vi "BRig_RT_panel_ExpStruct_v1,18.vi"(7 "input_setValues":bool, 11 "input_dataExp":u16[](array[numeric])) -> (3 "output_dataExp":u16[](array[numeric]))   [LabVIEW 2014]
panel:
  in  "DAB_flipLR_nTrial_opt":bool caption="Rewards\n\nTrials"
  in  "DAB_flipLR_nTrial":u16=100 caption="Flip Directionality\nAfter X trials" max=1000 step=1
  in  "I_L_nTrig_PerState":bool
  in  "I_Cue2":bool caption="Enable Cue2?\n\n\nENL2\n\nCue2 Audio\nCue2 LED"
  in  "T_Cue2_LED_max":u16=1000 caption="Max" min=5 max=5000 step=5
  in  "T_Cue2_LED_min":u16=1000 caption="Min" min=5 max=5000 step=5
  in  "T_Cue2_LED_step":u16=1000 caption="Penalty" min=1 max=10000 step=1
  in  "T_Cue2_Audio_max":u16=1000 caption="Max" min=5 max=5000 step=5
  in  "T_Cue2_Audio_min":u16=1000 caption="Min" min=5 max=5000 step=5
  in  "T_Cue2_Audio_step":u16=1000 caption="Penalty" min=1 max=10000 step=1
  in  "T_ENL2_step":u16=100 caption="Penalty" min=10 max=10000 step=10
  in  "T_ENL2_max":u16=1000 caption="Max" min=250 max=10000 step=250
  in  "T_ENL2_min":u16=1000 caption="Min" min=250 max=10000 step=250
  in  "ClosedLoop_LaserHold_l2":bool
  in  "ClosedLoop_LaserHold_l1":bool
  in  "FreeReward_Count2":u16 caption="# consecutive NonForcedError trials"
  in  "FreeReward_Count1":u16 caption="# consecutive ReBiasing trials"
  in  "FreeReward_Switch":bool caption="Give Reward If\nToo Many Errors"
  in  "T_CuePenalty":u16=1000 caption="Penalty" min=1 max=10000 step=1
  in  "T_ENLPenalty":u16=100 caption="Penalty" min=10 max=10000 step=10
  in  "LaserSwitch_Probability_L1":u16
  in  "LaserSwitch":u16(slide) max=3 step=1 scale=0.0..3.0
  in  "I_DAB":bool caption="NonSpecific\nLick Direction"
  in  "Tcycle_Reward_max_R":u16=1000 caption="Max" min=5 max=5000 step=5
  in  "Tcycle_Reward_min_R":u16=1000 caption="Min" min=5 max=5000 step=5
  in  "Tcycle_Reward_step_R":u16=1000 caption="Penalty" min=1 max=10000 step=1
  in  "Tcycle_Reward_max_L":u16=1000 caption="Max" min=5 max=5000 step=5
  in  "Tcycle_Reward_min_L":u16=1000 caption="Min" min=5 max=5000 step=5
  in  "Tcycle_Reward_step_L":u16=1000 caption="Penalty" min=1 max=10000 step=1
  in  "T_Cue_LED_max":u16=1000 caption="Max" min=5 max=5000 step=5
  in  "T_Cue_LED_min":u16=1000 caption="Min" min=5 max=5000 step=5
  in  "T_Cue_LED_step":u16=1000 caption="Penalty" min=1 max=10000 step=1
  in  "SolenoidProbability_L":u16=100 caption="Reward Time [ms]" min=1 max=1000 step=1
  in  "SolenoidProbability_R":u16=100 caption="Reward Time [ms]" min=1 max=1000 step=1
  in  "T_Cue_Audio_max":u16=1000 caption="Max" min=5 max=5000 step=5
  in  "T_Cue_Audio_min":u16=1000 caption="Min" min=5 max=5000 step=5
  in  "BUR_max":u16 caption="Max"
  in  "Tcycle_Timeout":u16=1000 caption="Timeout Time [ms]" min=10 max=10000 step=1
  in  "Tcycle_Wrong":u16=1000 caption="Penalty - Wrong Choice" min=10 max=10000 step=1
  in  "Tcycle_Selection":u16=1000 caption="Answer Time [ms]" min=1 max=10000 step=1
  in  "Tcycle_RewardPost":u16=1000 caption="Consumption Time [ms]" min=250 max=10000 step=250
  in  "TpB_Max_R":u16=4 caption="Max R" min=1 max=12 step=1
  in  "TpB_Min_R":u16=4 caption="Min R" min=1 max=12 step=1
  in  "TpB_Max_L":u16=4 caption="Max L" min=1 max=12 step=1
  in  "TpB_Min_L":u16=4 caption="Min L" min=1 max=12 step=1
  in  "BUR_min":u16 caption="Min"
  in  "TrialUntilReward":bool caption="Ignore Wrong\nSelections?"
  in  "T_Cue_Audio_step":u16=1000 caption="Penalty" min=1 max=10000 step=1
  in  "T_ENL_step":u16=100 caption="Penalty" min=10 max=10000 step=10
  in  "T_ENL_max":u16=1000 caption="Max" min=250 max=10000 step=250
  in  "T_ENL_min":u16=1000 caption="Min" min=250 max=10000 step=250
  # "Experiment Task Structure"
  # "Min            Max               Step        Penalty"
  # "(Laser1 or Laser2)\nLaser1 probability"
  # "Enforced\nNonLick"
  # "Cue Audio"
  # "(ClosedLoop Structure)"
  # "Hold Laser1"
  # "Hold Laser2"
  # "Cue LED"
  # "Allow Multiple Laser\nTriggers During\nENL and Cue?"
  # "Dual Armed Bandit"
  # "Selection"
  # "Reward - Dispense Water"
  # "Min            Max            StepSize"
  # "Left"
  # "Right"
  # "Count Reward Structure\n(0 = off)"
  # "Dispense Water Probability"
  # "%"
  # "Left"
  # "Right"
  # "%"
  # "Trial Per Block Structure \n               Left                        Right"
  # "Reward - Consumption"
  # "Penalty - Choice Timeout"
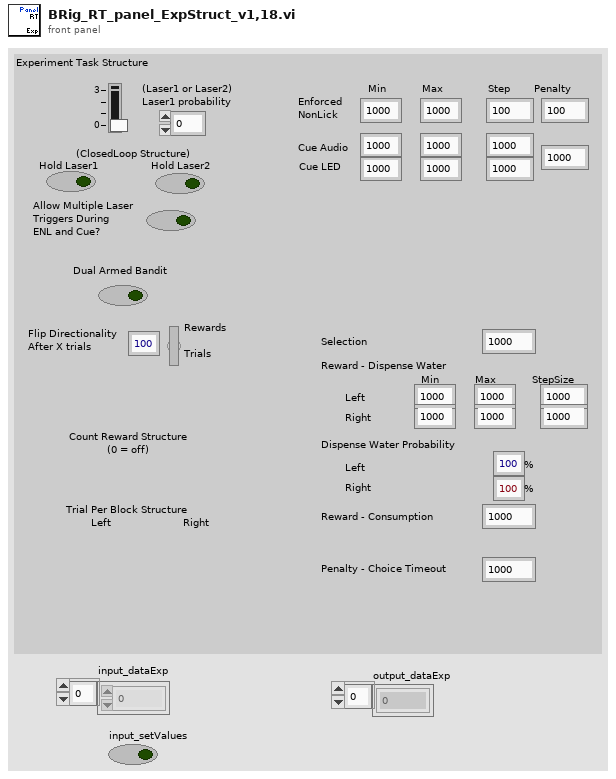
[diagram p1: front panel]
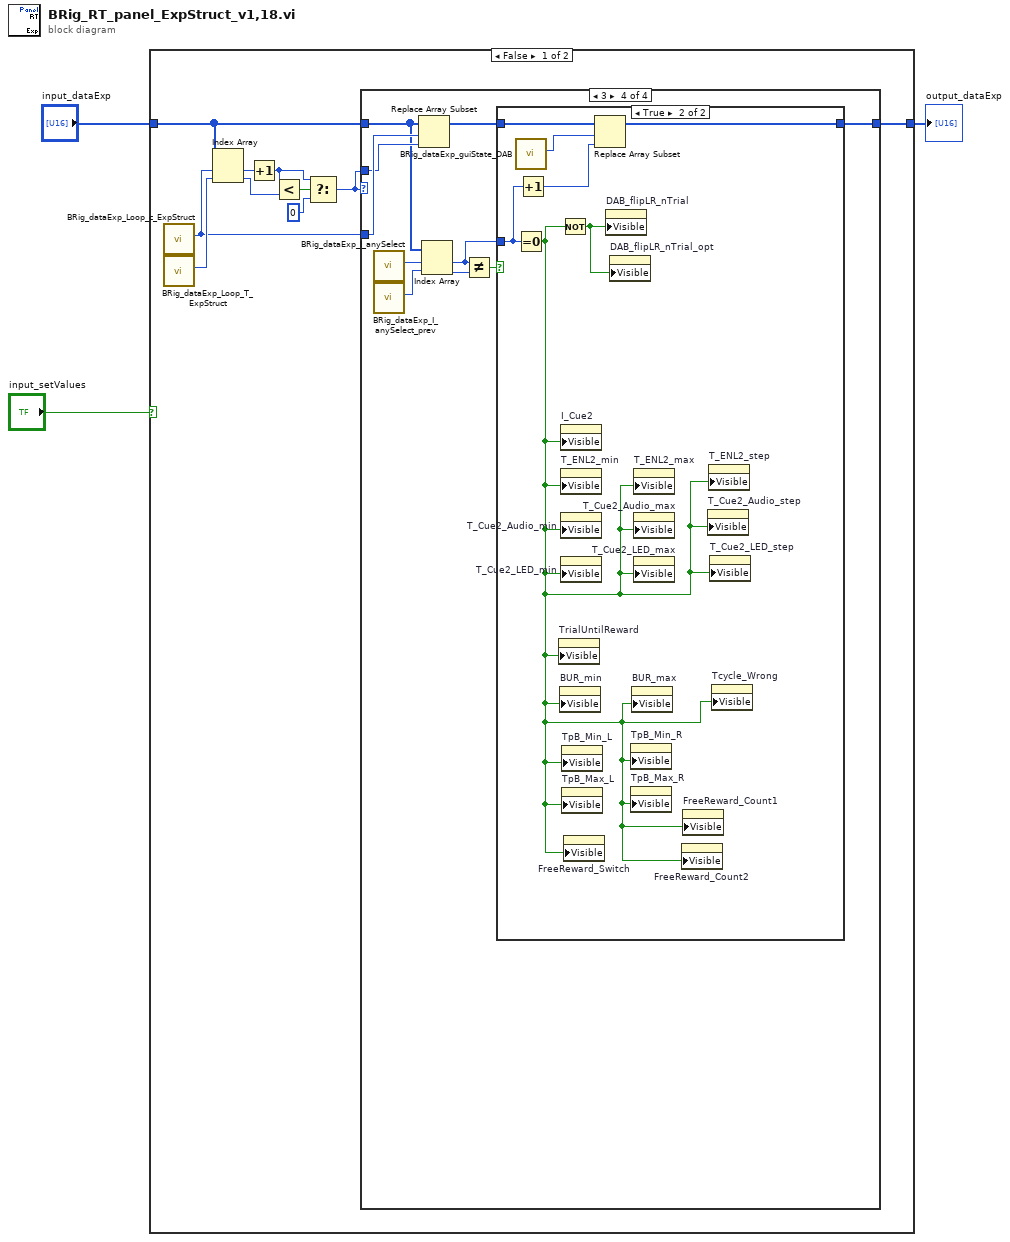
[diagram p0: block diagram]
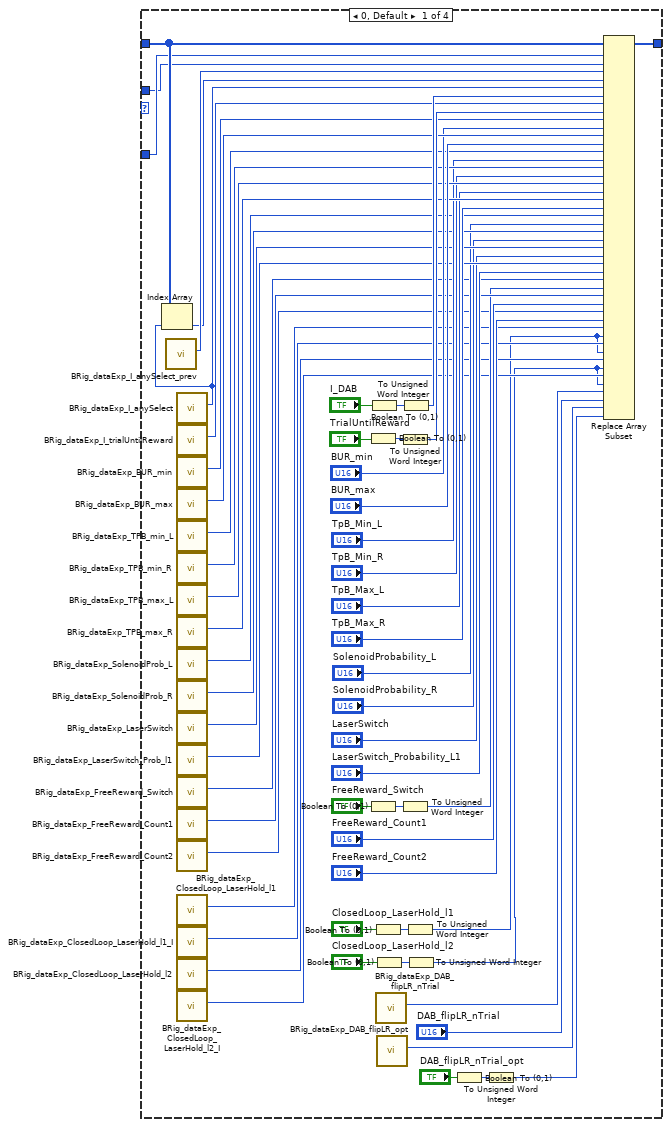
[diagram p2: hidden frame]
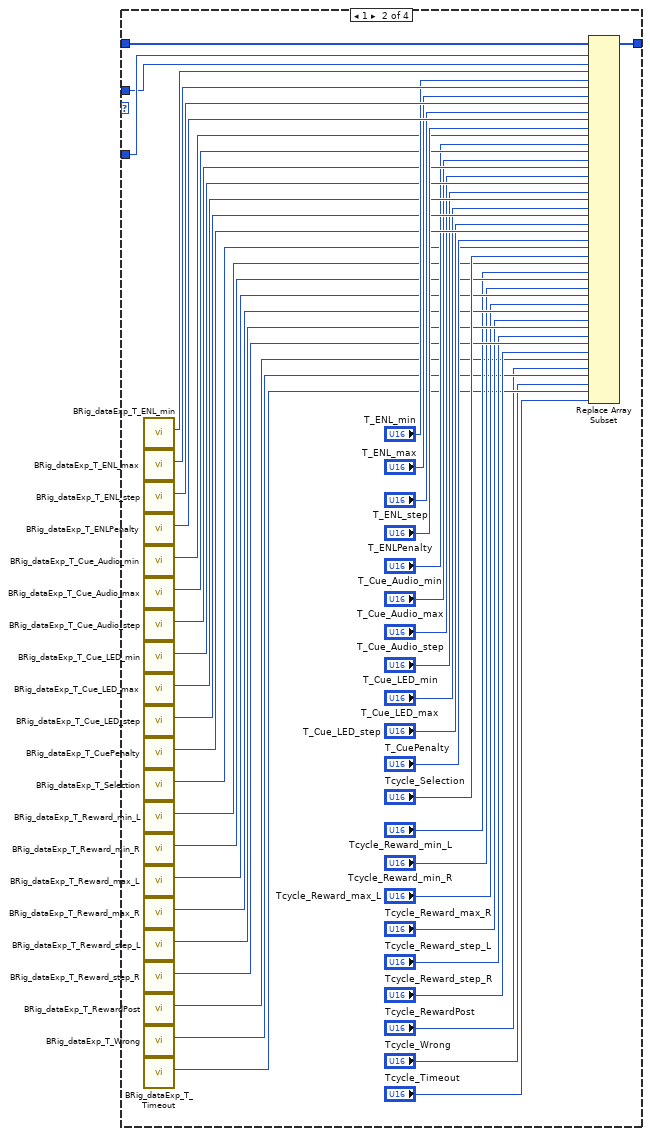
[diagram p3: hidden frame]
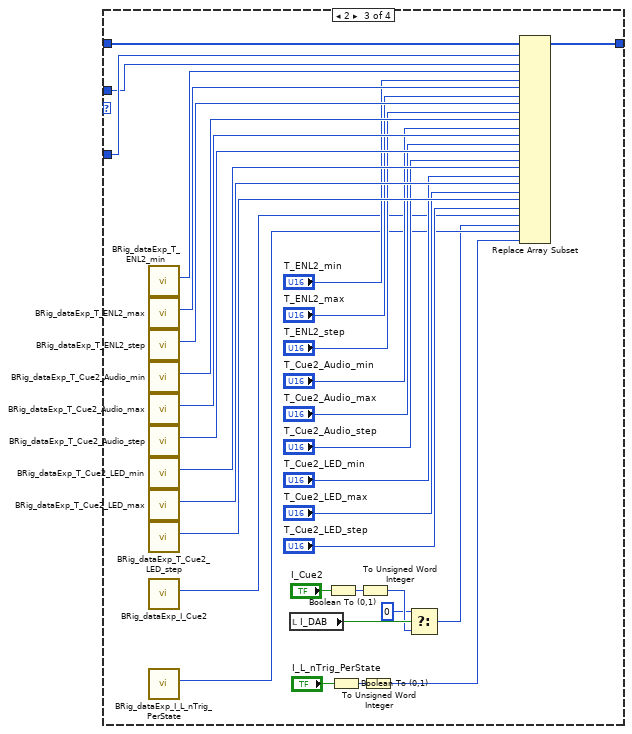
[diagram p4: hidden frame]
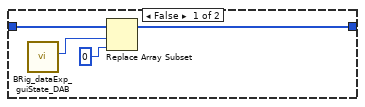
[diagram p5: hidden frame]
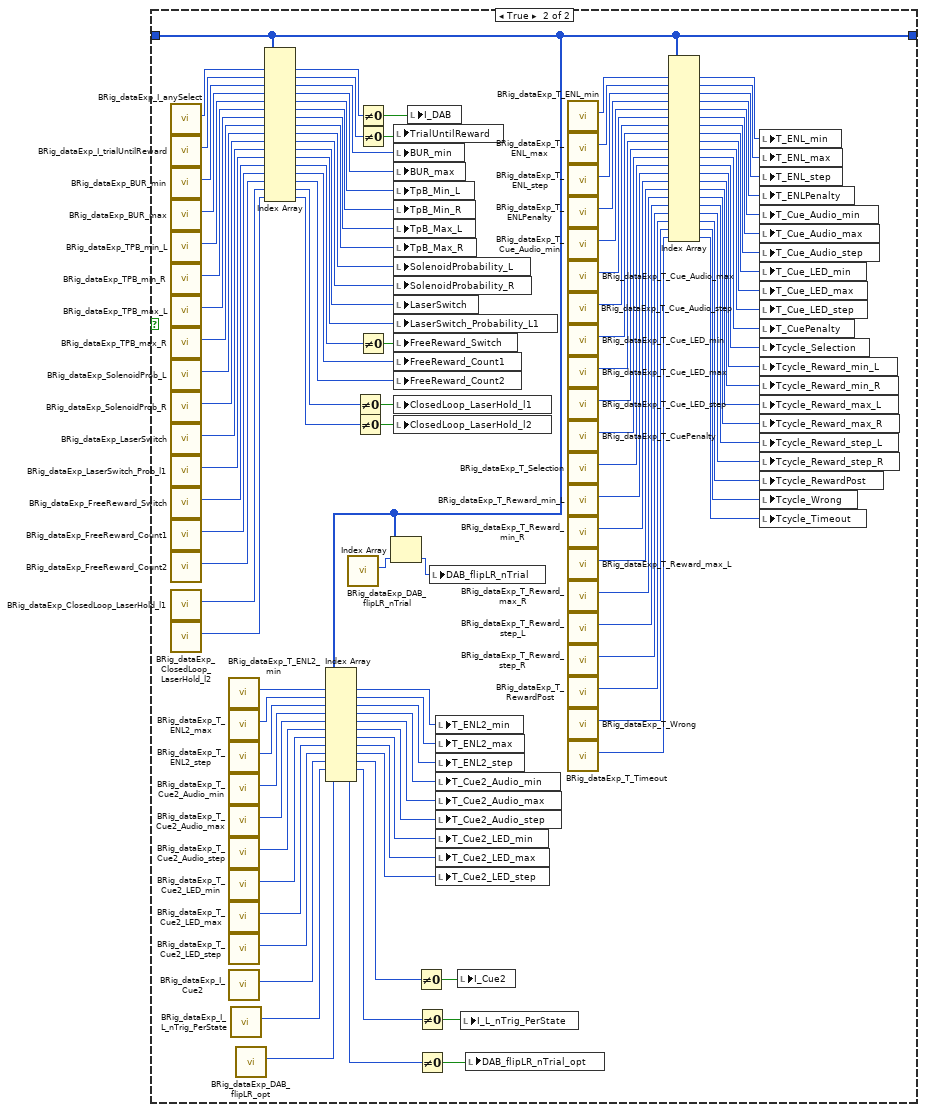
[diagram p6: hidden frame]
diagram:
  n1 = case shown="False" "input_setValues" {
    tunnel: [w13 w177] -> w3
    tunnel: "input_dataExp" -> [w12 w177]
    frame False {
      n2 = call "BRig_dataExp_Loop_c_ExpStruct.vi"() -> ("output_Loop_c_ExpStruct"=w6:i32)  [unwired: 11 in]
      n3 = call "BRig_dataExp_Loop_T_ExpStruct.vi"() -> ("output_Loop_T_ExpStruct"=w11:i32)  [unwired: 11 in]
      n4 = Index Array(array=w12, index #1=w6, index #2=w11) -> (element #1=w10:u16, element #2=w9:u16)
      n5 = Increment(x=w10) -> (x+1=w5:u16)
      n6 = Less?(x=w5, y=w9) -> (x < y?=w8:bool)
      n7 = Select(t=w5, s=w8, f=u16 0) -> (s? t:f=w4:u16)
      n8 = case shown="3" w4 {
        tunnel: w12 -> [w23 w117 w150 w157]
        tunnel: [w71 w116 w149 w152] -> w13
        tunnel: w6 -> [w21 w115 w148 w160]
        tunnel: w4 -> [w20 w114 w147 w159]
        frame 0, Default {
          n9 = call "BRig_dataExp_I_anySelect_prev.vi"() -> ("output_I_anySelect_prev"=w19:i32)  [unwired: 11 in]
          n10 = call "BRig_dataExp_I_anySelect.vi"() -> ("output_I_anySelect"=w22:i32)  [unwired: 11 in]
          n11 = Index Array(array=w23, index=w22) -> (element=w18:u16)
          n12 = call "BRig_dataExp_I_trialUntilReward.vi"() -> ("output_I_trialUntilReward"=w67:i32)  [unwired: 11 in]
          n13 = call "BRig_dataExp_BUR_min.vi"() -> ("output_BUR_min"=w63:i32)  [unwired: 11 in]
          n14 = call "BRig_dataExp_BUR_max.vi"() -> ("output_BUR_max"=w62:i32)  [unwired: 11 in]
          n15 = call "BRig_dataExp_TPB_min_L.vi"() -> ("output_TPB_min_L"=w59:i32)  [unwired: 11 in]
          n16 = call "BRig_dataExp_TPB_min_R.vi"() -> ("output_TPB_min_R"=w58:i32)  [unwired: 11 in]
          n17 = call "BRig_dataExp_TPB_max_L.vi"() -> ("output_TPB_max_L"=w57:i32)  [unwired: 11 in]
          n18 = call "BRig_dataExp_TPB_max_R.vi"() -> ("output_TPB_max_R"=w56:i32)  [unwired: 11 in]
          n19 = call "BRig_dataExp_SolenoidProb_L.vi"() -> ("output_SolenoidProbability_L"=w51:i32)  [unwired: 11 in]
          n20 = call "BRig_dataExp_SolenoidProb_R.vi"() -> ("output_SolenoidProbability_R"=w50:i32)  [unwired: 11 in]
          n21 = call "BRig_dataExp_LaserSwitch.vi"() -> ("output_LaserSwitch"=w49:i32)  [unwired: 11 in]
          n22 = call "BRig_dataExp_LaserSwitch_Prob_l1.vi"() -> ("output_LaserSwitch_Probability_L1"=w48:i32)  [unwired: 11 in]
          n23 = call "BRig_dataExp_FreeReward_Switch.vi"() -> ("output_FreeReward_Switch"=w41:i32)  [unwired: 11 in]
          n24 = call "BRig_dataExp_FreeReward_Count1.vi"() -> ("output_FreeReward_Count"=w40:i32)  [unwired: 11 in]
          n25 = call "BRig_dataExp_FreeReward_Count2.vi"() -> ("output_FreeReward_Count"=w37:i32)  [unwired: 11 in]
          n26 = call "BRig_dataExp_ClosedLoop_LaserHold_l1.vi"() -> ("output_CloseLoop_LaserHold_l1"=w35:i32)  [unwired: 11 in]
          n27 = call "BRig_dataExp_ClosedLoop_LaserHold_l1_I.vi"() -> ("output_CloseLoop_LaserHold_l1_I"=w34:i32)  [unwired: 11 in]
          n28 = call "BRig_dataExp_ClosedLoop_LaserHold_l2.vi"() -> ("output_CloseLoop_LaserHold_l2"=w33:i32)  [unwired: 11 in]
          n29 = call "BRig_dataExp_ClosedLoop_LaserHold_l2_I.vi"() -> ("output_CloseLoop_LaserHold_l2_I"=w32:i32)  [unwired: 11 in]
          n30 = Boolean To (0,1)(Boolean="TrialUntilReward") -> (0, 1=w66:i16)
          n31 = Boolean To (0,1)(Boolean="FreeReward_Switch") -> (0, 1=w43:i16)
          n32 = Boolean To (0,1)(Boolean="I_DAB") -> (0, 1=w69:i16)
          n33 = Boolean To (0,1)(Boolean="ClosedLoop_LaserHold_l1") -> (0, 1=w31:i16)
          n34 = Boolean To (0,1)(Boolean="ClosedLoop_LaserHold_l2") -> (0, 1=w29:i16)
          n35 = call "BRig_dataExp_DAB_flipLR_nTrial.vi"() -> ("output_DAB_flipLR_nTrial"=w25:i32)  [unwired: 11 in]
          n36 = call "BRig_dataExp_DAB_flipLR_opt.vi"() -> ("output_DAB_flipLR_opt"=w17:i32)  [unwired: 11 in]
          n37 = To Unsigned Word Integer(number=w66) -> (unsigned 16bit integer=w64:u16)
          n38 = To Unsigned Word Integer(number=w43) -> (unsigned 16bit integer=w39:u16)
          n39 = To Unsigned Word Integer(number=w69) -> (unsigned 16bit integer=w68:u16)
          n40 = To Unsigned Word Integer(number=w31) -> (unsigned 16bit integer=w27:u16)
          n41 = To Unsigned Word Integer(number=w29) -> (unsigned 16bit integer=w26:u16)
          n42 = Boolean To (0,1)(Boolean="DAB_flipLR_nTrial_opt") -> (0, 1=w16:i16)
          n43 = To Unsigned Word Integer(number=w16) -> (unsigned 16bit integer=w14:u16)
          n44 = Replace Array Subset(array=w23, new element #1=w20, index #1=w21, new element #2=w18, index #2=w19, new element #3=w68, index #3=w22, new element #4=w64, index #4=w67, new element #5="BUR_min", index #5=w63, new element #6="BUR_max", index #6=w62, new element #7="TpB_Min_L", index #7=w59, new element #8="TpB_Min_R", index #8=w58, new element #9="TpB_Max_L", index #9=w57, new element #10="TpB_Max_R", index #10=w56, new element #11="SolenoidProbability_L", index #11=w51, new element #12="SolenoidProbability_R", index #12=w50, new element #13="LaserSwitch", index #13=w49, new element #14="LaserSwitch_Probability_L1", index #14=w48, new element #15=w39, index #15=w41, new element #16="FreeReward_Count1", index #16=w40, new element #17="FreeReward_Count2", index #17=w37, new element #18=w27, index #18=w35, new element #19=w27, index #19=w34, new element #20=w26, index #20=w33, new element #21=w26, index #21=w32, new element #22="DAB_flipLR_nTrial", index #22=w25, new element #23=w14, index #23=w17) -> (w71:u16[])
        }
        frame 1 {
          n45 = call "BRig_dataExp_T_ENL_min.vi"() -> ("output_T_ENL_min"=w113:i32)  [unwired: 11 in]
          n46 = call "BRig_dataExp_T_ENL_max.vi"() -> ("output_T_ENL_max"=w112:i32)  [unwired: 11 in]
          n47 = call "BRig_dataExp_T_ENL_step.vi"() -> ("output_T_ENL_step"=w111:i32)  [unwired: 11 in]
          n48 = call "BRig_dataExp_T_ENLPenalty.vi"() -> ("output_ENL_penalty"=w110:i32)  [unwired: 11 in]
          n49 = call "BRig_dataExp_T_Cue_Audio_min.vi"() -> ("output_T_Cue_Audio_min"=w105:i32)  [unwired: 11 in]
          n50 = call "BRig_dataExp_T_Cue_Audio_max.vi"() -> ("output_T_Cue_Audio_max"=w104:i32)  [unwired: 11 in]
          n51 = call "BRig_dataExp_T_Cue_Audio_step.vi"() -> ("output_T_Cue_Audio_step"=w103:i32)  [unwired: 11 in]
          n52 = call "BRig_dataExp_T_Cue_LED_min.vi"() -> ("output_T_Cue_LED_min"=w102:i32)  [unwired: 11 in]
          n53 = call "BRig_dataExp_T_Cue_LED_max.vi"() -> ("output_T_Cue_LED_max"=w101:i32)  [unwired: 11 in]
          n54 = call "BRig_dataExp_T_Cue_LED_step.vi"() -> ("output_T_Cue_LED_step"=w100:i32)  [unwired: 11 in]
          n55 = call "BRig_dataExp_T_CuePenalty.vi"() -> ("output_T_CuePenalty"=w99:i32)  [unwired: 11 in]
          n56 = call "BRig_dataExp_T_Selection.vi"() -> ("output_T_Selection"=w91:i32)  [unwired: 11 in]
          n57 = call "BRig_dataExp_T_Reward_min_L.vi"() -> ("output_Tcycle_Reward_min_L"=w89:i32)  [unwired: 11 in]
          n58 = call "BRig_dataExp_T_Reward_min_R.vi"() -> ("output_T_Reward_min_R"=w88:i32)  [unwired: 11 in]
          n59 = call "BRig_dataExp_T_Reward_max_L.vi"() -> ("output_T_Reward_max_L"=w87:i32)  [unwired: 11 in]
          n60 = call "BRig_dataExp_T_Reward_max_R.vi"() -> ("output_T_Reward_max_R"=w86:i32)  [unwired: 11 in]
          n61 = call "BRig_dataExp_T_Reward_step_L.vi"() -> ("output_T_Reward_step_L"=w85:i32)  [unwired: 11 in]
          n62 = call "BRig_dataExp_T_Reward_step_R.vi"() -> ("output_T_Reward_step_R"=w84:i32)  [unwired: 11 in]
          n63 = call "BRig_dataExp_T_RewardPost.vi"() -> ("output_T_RewardPost"=w77:i32)  [unwired: 11 in]
          n64 = call "BRig_dataExp_T_Wrong.vi"() -> ("output_T_Wrong"=w76:i32)  [unwired: 11 in]
          n65 = call "BRig_dataExp_T_Timeout.vi"() -> ("output_T_Timeout"=w75:i32)  [unwired: 11 in]
          n66 = Replace Array Subset(array=w117, new element #1=w114, index #1=w115, new element #2="T_ENL_min", index #2=w113, new element #3="T_ENL_max", index #3=w112, new element #4="T_ENL_step", index #4=w111, new element #5="T_ENLPenalty", index #5=w110, new element #6="T_Cue_Audio_min", index #6=w105, new element #7="T_Cue_Audio_max", index #7=w104, new element #8="T_Cue_Audio_step", index #8=w103, new element #9="T_Cue_LED_min", index #9=w102, new element #10="T_Cue_LED_max", index #10=w101, new element #11="T_Cue_LED_step", index #11=w100, new element #12="T_CuePenalty", index #12=w99, new element #13="Tcycle_Selection", index #13=w91, new element #14="Tcycle_Reward_min_L", index #14=w89, new element #15="Tcycle_Reward_min_R", index #15=w88, new element #16="Tcycle_Reward_max_L", index #16=w87, new element #17="Tcycle_Reward_max_R", index #17=w86, new element #18="Tcycle_Reward_step_L", index #18=w85, new element #19="Tcycle_Reward_step_R", index #19=w84, new element #20="Tcycle_RewardPost", index #20=w77, new element #21="Tcycle_Wrong", index #21=w76, new element #22="Tcycle_Timeout", index #22=w75) -> (w116:u16[])
        }
        frame 2 {
          n67 = call "BRig_dataExp_T_ENL2_min.vi"() -> ("output_T_ENL2_min"=w146:i32)  [unwired: 11 in]
          n68 = call "BRig_dataExp_T_ENL2_max.vi"() -> ("output_T_ENL2_max"=w145:i32)  [unwired: 11 in]
          n69 = call "BRig_dataExp_T_ENL2_step.vi"() -> ("output_T_ENL2_step"=w144:i32)  [unwired: 11 in]
          n70 = call "BRig_dataExp_T_Cue2_Audio_min.vi"() -> ("output_T_Cue2_Audio_min"=w143:i32)  [unwired: 11 in]
          n71 = call "BRig_dataExp_T_Cue2_Audio_max.vi"() -> ("output_T_Cue2_Audio_max"=w142:i32)  [unwired: 11 in]
          n72 = call "BRig_dataExp_T_Cue2_Audio_step.vi"() -> ("output_T_Cue2_Audio_step"=w141:i32)  [unwired: 11 in]
          n73 = call "BRig_dataExp_T_Cue2_LED_min.vi"() -> ("output_T_Cue2_LED_min"=w140:i32)  [unwired: 11 in]
          n74 = call "BRig_dataExp_T_Cue2_LED_max.vi"() -> ("output_T_Cue2_LED_max"=w139:i32)  [unwired: 11 in]
          n75 = call "BRig_dataExp_T_Cue2_LED_step.vi"() -> ("output_T_Cue2_LED_step"=w138:i32)  [unwired: 11 in]
          n76 = call "BRig_dataExp_I_Cue2.vi"() -> ("output_I_Cue2"=w128:i32)  [unwired: 11 in]
          n77 = call "BRig_dataExp_I_L_nTrig_PerState.vi"() -> ("output_I_L_nTrig_PerState"=w125:i32)  [unwired: 11 in]
          n78 = local read "I_DAB"() -> (w121:bool)
          n79 = Boolean To (0,1)(Boolean="I_Cue2") -> (0, 1=w126:i16)
          n80 = Boolean To (0,1)(Boolean="I_L_nTrig_PerState") -> (0, 1=w124:i16)
          n81 = To Unsigned Word Integer(number=w126) -> (unsigned 16bit integer=w119:u16)
          n82 = To Unsigned Word Integer(number=w124) -> (unsigned 16bit integer=w122:u16)
          n83 = Select(t=u16 0 ("f"), s=w121, f=w119) -> (s? t:f=w120:u16)
          n84 = Replace Array Subset(array=w150, new element #1=w147, index #1=w148, new element #2="T_ENL2_min", index #2=w146, new element #3="T_ENL2_max", index #3=w145, new element #4="T_ENL2_step", index #4=w144, new element #5="T_Cue2_Audio_min", index #5=w143, new element #6="T_Cue2_Audio_max", index #6=w142, new element #7="T_Cue2_Audio_step", index #7=w141, new element #8="T_Cue2_LED_min", index #8=w140, new element #9="T_Cue2_LED_max", index #9=w139, new element #10="T_Cue2_LED_step", index #10=w138, new element #11=w120, index #11=w128, new element #12=w122, index #12=w125) -> (w149:u16[])
        }
        frame 3 {
          n85 = call "BRig_dataExp_I_anySelect.vi"() -> ("output_I_anySelect"=w158:i32)  [unwired: 11 in]
          n86 = call "BRig_dataExp_I_anySelect_prev.vi"() -> ("output_I_anySelect_prev"=w156:i32)  [unwired: 11 in]
          n87 = Replace Array Subset(array=w157, new element=w159, index=w160) -> (w153:u16[])
          n88 = Index Array(array=w157, index #1=w158, index #2=w156) -> (element #1=w151:u16, element #2=w155:u16)
          n89 = Not Equal?(x=w151, y=w155) -> (x != y?=w154:bool)
          n90 = case shown="True" w154 {
            tunnel: w153 -> [w164 w171]
            tunnel: [w163 w170] -> w152
            tunnel: w151 -> [_ w167]
            frame False {
              n91 = call "BRig_dataExp_guiState_DAB.vi"() -> ("output_guiState_DAB"=w162:i32)  [unwired: 11 in]
              n92 = Replace Array Subset(array=w164, new element=u16 0 ("new element/subarray"), index=w162) -> (w163:u16[])
            }
            frame True {
              n93 = call "BRig_dataExp_guiState_DAB.vi"() -> ("output_guiState_DAB"=w169:i32)  [unwired: 11 in]
              n94 = Equal To 0?(x=w167) -> (x = 0?=w166:bool)
              n95 = Increment(x=w167) -> (x+1=w168:u16)
              n96 = property on="TrialUntilReward" class="Bool (strict)"("Visible"=w166) -> ()  [unwired: 2 in, 2 out]
              n97 = Not(x=w166) -> (.not. x?=w165:bool)
              n98 = property on="BUR_min" class="DigNum (strict)"("Visible"=w166) -> ()  [unwired: 2 in, 2 out]
              n99 = property on="I_Cue2" class="Bool (strict)"("Visible"=w166) -> ()  [unwired: 2 in, 2 out]
              n100 = property on="T_ENL2_min" class="DigNum (strict)"("Visible"=w166) -> ()  [unwired: 2 in, 2 out]
              n101 = property on="T_Cue2_Audio_min" class="DigNum (strict)"("Visible"=w166) -> ()  [unwired: 2 in, 2 out]
              n102 = property on="T_Cue2_LED_min" class="DigNum (strict)"("Visible"=w166) -> ()  [unwired: 2 in, 2 out]
              n103 = property on="TpB_Min_L" class="DigNum (strict)"("Visible"=w166) -> ()  [unwired: 2 in, 2 out]
              n104 = property on="TpB_Max_L" class="DigNum (strict)"("Visible"=w166) -> ()  [unwired: 2 in, 2 out]
              n105 = property on="FreeReward_Switch" class="Bool (strict)"("Visible"=w166) -> ()  [unwired: 2 in, 2 out]
              n106 = Replace Array Subset(array=w171, new element=w168, index=w169) -> (w170:u16[])
              n107 = property on="DAB_flipLR_nTrial" class="DigNum (strict)"("Visible"=w165) -> ()  [unwired: 2 in, 2 out]
              n108 = property on="DAB_flipLR_nTrial_opt" class="Bool (strict)"("Visible"=w165) -> ()  [unwired: 2 in, 2 out]
              n109 = property on="TpB_Min_R" class="DigNum (strict)"("Visible"=w166) -> ()  [unwired: 2 in, 2 out]
              n110 = property on="TpB_Max_R" class="DigNum (strict)"("Visible"=w166) -> ()  [unwired: 2 in, 2 out]
              n111 = property on="BUR_max" class="DigNum (strict)"("Visible"=w166) -> ()  [unwired: 2 in, 2 out]
              n112 = property on="T_ENL2_max" class="DigNum (strict)"("Visible"=w166) -> ()  [unwired: 2 in, 2 out]
              n113 = property on="T_Cue2_Audio_max" class="DigNum (strict)"("Visible"=w166) -> ()  [unwired: 2 in, 2 out]
              n114 = property on="T_Cue2_LED_max" class="DigNum (strict)"("Visible"=w166) -> ()  [unwired: 2 in, 2 out]
              n115 = property on="FreeReward_Count2" class="DigNum (strict)"("Visible"=w166) -> ()  [unwired: 2 in, 2 out]
              n116 = property on="FreeReward_Count1" class="DigNum (strict)"("Visible"=w166) -> ()  [unwired: 2 in, 2 out]
              n117 = property on="T_Cue2_Audio_step" class="DigNum (strict)"("Visible"=w166) -> ()  [unwired: 2 in, 2 out]
              n118 = property on="T_ENL2_step" class="DigNum (strict)"("Visible"=w166) -> ()  [unwired: 2 in, 2 out]
              n119 = property on="T_Cue2_LED_step" class="DigNum (strict)"("Visible"=w166) -> ()  [unwired: 2 in, 2 out]
              n120 = property on="Tcycle_Wrong" class="DigNum (strict)"("Visible"=w166) -> ()  [unwired: 2 in, 2 out]
            }
          }
        }
      }
    }
    frame True {
      n121 = call "BRig_dataExp_I_anySelect.vi"() -> ("output_I_anySelect"=w282:i32)  [unwired: 11 in]
      n122 = call "BRig_dataExp_I_trialUntilReward.vi"() -> ("output_I_trialUntilReward"=w281:i32)  [unwired: 11 in]
      n123 = call "BRig_dataExp_BUR_min.vi"() -> ("output_BUR_min"=w280:i32)  [unwired: 11 in]
      n124 = call "BRig_dataExp_BUR_max.vi"() -> ("output_BUR_max"=w279:i32)  [unwired: 11 in]
      n125 = call "BRig_dataExp_TPB_min_L.vi"() -> ("output_TPB_min_L"=w278:i32)  [unwired: 11 in]
      n126 = call "BRig_dataExp_TPB_min_R.vi"() -> ("output_TPB_min_R"=w277:i32)  [unwired: 11 in]
      n127 = call "BRig_dataExp_TPB_max_L.vi"() -> ("output_TPB_max_L"=w276:i32)  [unwired: 11 in]
      n128 = call "BRig_dataExp_TPB_max_R.vi"() -> ("output_TPB_max_R"=w275:i32)  [unwired: 11 in]
      n129 = call "BRig_dataExp_SolenoidProb_L.vi"() -> ("output_SolenoidProbability_L"=w274:i32)  [unwired: 11 in]
      n130 = call "BRig_dataExp_SolenoidProb_R.vi"() -> ("output_SolenoidProbability_R"=w273:i32)  [unwired: 11 in]
      n131 = call "BRig_dataExp_LaserSwitch.vi"() -> ("output_LaserSwitch"=w272:i32)  [unwired: 11 in]
      n132 = call "BRig_dataExp_LaserSwitch_Prob_l1.vi"() -> ("output_LaserSwitch_Probability_L1"=w271:i32)  [unwired: 11 in]
      n133 = call "BRig_dataExp_FreeReward_Switch.vi"() -> ("output_FreeReward_Switch"=w270:i32)  [unwired: 11 in]
      n134 = call "BRig_dataExp_FreeReward_Count1.vi"() -> ("output_FreeReward_Count"=w269:i32)  [unwired: 11 in]
      n135 = call "BRig_dataExp_FreeReward_Count2.vi"() -> ("output_FreeReward_Count"=w209:i32)  [unwired: 11 in]
      n136 = call "BRig_dataExp_ClosedLoop_LaserHold_l1.vi"() -> ("output_CloseLoop_LaserHold_l1"=w207:i32)  [unwired: 11 in]
      n137 = call "BRig_dataExp_ClosedLoop_LaserHold_l2.vi"() -> ("output_CloseLoop_LaserHold_l2"=w206:i32)  [unwired: 11 in]
      n138 = call "BRig_dataExp_T_ENL2_min.vi"() -> ("output_T_ENL2_min"=w201:i32)  [unwired: 11 in]
      n139 = call "BRig_dataExp_T_ENL2_max.vi"() -> ("output_T_ENL2_max"=w200:i32)  [unwired: 11 in]
      n140 = call "BRig_dataExp_T_ENL2_step.vi"() -> ("output_T_ENL2_step"=w199:i32)  [unwired: 11 in]
      n141 = call "BRig_dataExp_T_Cue2_Audio_min.vi"() -> ("output_T_Cue2_Audio_min"=w198:i32)  [unwired: 11 in]
      n142 = call "BRig_dataExp_T_Cue2_Audio_max.vi"() -> ("output_T_Cue2_Audio_max"=w197:i32)  [unwired: 11 in]
      n143 = call "BRig_dataExp_T_Cue2_Audio_step.vi"() -> ("output_T_Cue2_Audio_step"=w196:i32)  [unwired: 11 in]
      n144 = call "BRig_dataExp_T_Cue2_LED_min.vi"() -> ("output_T_Cue2_LED_min"=w195:i32)  [unwired: 11 in]
      n145 = call "BRig_dataExp_T_Cue2_LED_max.vi"() -> ("output_T_Cue2_LED_max"=w194:i32)  [unwired: 11 in]
      n146 = call "BRig_dataExp_T_Cue2_LED_step.vi"() -> ("output_T_Cue2_LED_step"=w193:i32)  [unwired: 11 in]
      n147 = call "BRig_dataExp_I_Cue2.vi"() -> ("output_I_Cue2"=w183:i32)  [unwired: 11 in]
      n148 = call "BRig_dataExp_I_L_nTrig_PerState.vi"() -> ("output_I_L_nTrig_PerState"=w180:i32)  [unwired: 11 in]
      n149 = call "BRig_dataExp_DAB_flipLR_opt.vi"() -> ("output_DAB_flipLR_opt"=w174:i32)  [unwired: 11 in]
      n150 = Index Array(array=w177, index #1=w282, index #2=w281, index #3=w280, index #4=w279, index #5=w278, index #6=w277, index #7=w276, index #8=w275, index #9=w274, index #10=w273, index #11=w272, index #12=w271, index #13=w270, index #14=w269, index #15=w209, index #16=w207, index #17=w206) -> (element #1=w265:u16, element #2=w264:u16, element #3=w263:u16, element #4=w262:u16, element #5=w261:u16, element #6=w260:u16, element #7=w259:u16, element #8=w258:u16, element #9=w257:u16, element #10=w256:u16, element #11=w255:u16, element #12=w254:u16, element #13=w253:u16, element #14=w252:u16, element #15=w208:u16, element #16=w203:u16, element #17=w202:u16)
      n151 = Index Array(array=w177, index #1=w201, index #2=w200, index #3=w199, index #4=w198, index #5=w197, index #6=w196, index #7=w195, index #8=w194, index #9=w193, index #10=w183, index #11=w180, index #12=w174) -> (element #1=w192:u16, element #2=w191:u16, element #3=w190:u16, element #4=w189:u16, element #5=w188:u16, element #6=w187:u16, element #7=w186:u16, element #8=w185:u16, element #9=w184:u16, element #10=w181:u16, element #11=w179:u16, element #12=w173:u16)
      n152 = call "BRig_dataExp_DAB_flipLR_nTrial.vi"() -> ("output_DAB_flipLR_nTrial"=w176:i32)  [unwired: 11 in]
      n153 = Not Equal To 0?(x=w203) -> (x != 0?=w205:bool)
      n154 = Not Equal To 0?(x=w202) -> (x != 0?=w204:bool)
      n155 = Not Equal To 0?(x=w265) -> (x != 0?=w268:bool)
      n156 = Not Equal To 0?(x=w264) -> (x != 0?=w267:bool)
      n157 = Not Equal To 0?(x=w253) -> (x != 0?=w266:bool)
      n158 = Index Array(array=w177, index=w176) -> (element=w175:u16)
      n159 = local write "TrialUntilReward"(w267) -> ()
      n160 = local write "BUR_min"(w263) -> ()
      n161 = local write "BUR_max"(w262) -> ()
      n162 = local write "TpB_Min_L"(w261) -> ()
      n163 = local write "TpB_Min_R"(w260) -> ()
      n164 = local write "TpB_Max_L"(w259) -> ()
      n165 = local write "TpB_Max_R"(w258) -> ()
      n166 = local write "SolenoidProbability_L"(w257) -> ()
      n167 = local write "SolenoidProbability_R"(w256) -> ()
      n168 = local write "LaserSwitch"(w255) -> ()
      n169 = local write "LaserSwitch_Probability_L1"(w254) -> ()
      n170 = local write "FreeReward_Switch"(w266) -> ()
      n171 = local write "FreeReward_Count1"(w252) -> ()
      n172 = local write "FreeReward_Count2"(w208) -> ()
      n173 = local write "ClosedLoop_LaserHold_l1"(w205) -> ()
      n174 = local write "ClosedLoop_LaserHold_l2"(w204) -> ()
      n175 = local write "I_DAB"(w268) -> ()
      n176 = Not Equal To 0?(x=w181) -> (x != 0?=w182:bool)
      n177 = Not Equal To 0?(x=w179) -> (x != 0?=w178:bool)
      n178 = Not Equal To 0?(x=w173) -> (x != 0?=w172:bool)
      n179 = local write "DAB_flipLR_nTrial"(w175) -> ()
      n180 = local write "T_ENL2_min"(w192) -> ()
      n181 = local write "T_ENL2_max"(w191) -> ()
      n182 = local write "T_ENL2_step"(w190) -> ()
      n183 = local write "T_Cue2_Audio_min"(w189) -> ()
      n184 = local write "T_Cue2_Audio_max"(w188) -> ()
      n185 = local write "T_Cue2_Audio_step"(w187) -> ()
      n186 = local write "T_Cue2_LED_min"(w186) -> ()
      n187 = local write "T_Cue2_LED_max"(w185) -> ()
      n188 = local write "T_Cue2_LED_step"(w184) -> ()
      n189 = local write "I_Cue2"(w182) -> ()
      n190 = local write "I_L_nTrig_PerState"(w178) -> ()
      n191 = local write "DAB_flipLR_nTrial_opt"(w172) -> ()
      n192 = call "BRig_dataExp_T_ENL_min.vi"() -> ("output_T_ENL_min"=w251:i32)  [unwired: 11 in]
      n193 = call "BRig_dataExp_T_ENL_max.vi"() -> ("output_T_ENL_max"=w250:i32)  [unwired: 11 in]
      n194 = call "BRig_dataExp_T_ENL_step.vi"() -> ("output_T_ENL_step"=w249:i32)  [unwired: 11 in]
      n195 = call "BRig_dataExp_T_ENLPenalty.vi"() -> ("output_ENL_penalty"=w248:i32)  [unwired: 11 in]
      n196 = call "BRig_dataExp_T_Cue_Audio_min.vi"() -> ("output_T_Cue_Audio_min"=w247:i32)  [unwired: 11 in]
      n197 = call "BRig_dataExp_T_Cue_Audio_max.vi"() -> ("output_T_Cue_Audio_max"=w246:i32)  [unwired: 11 in]
      n198 = call "BRig_dataExp_T_Cue_Audio_step.vi"() -> ("output_T_Cue_Audio_step"=w245:i32)  [unwired: 11 in]
      n199 = call "BRig_dataExp_T_Cue_LED_min.vi"() -> ("output_T_Cue_LED_min"=w244:i32)  [unwired: 11 in]
      n200 = call "BRig_dataExp_T_Cue_LED_max.vi"() -> ("output_T_Cue_LED_max"=w243:i32)  [unwired: 11 in]
      n201 = call "BRig_dataExp_T_Cue_LED_step.vi"() -> ("output_T_Cue_LED_step"=w242:i32)  [unwired: 11 in]
      n202 = call "BRig_dataExp_T_CuePenalty.vi"() -> ("output_T_CuePenalty"=w241:i32)  [unwired: 11 in]
      n203 = call "BRig_dataExp_T_Selection.vi"() -> ("output_T_Selection"=w240:i32)  [unwired: 11 in]
      n204 = call "BRig_dataExp_T_Reward_min_L.vi"() -> ("output_Tcycle_Reward_min_L"=w239:i32)  [unwired: 11 in]
      n205 = call "BRig_dataExp_T_Reward_min_R.vi"() -> ("output_T_Reward_min_R"=w238:i32)  [unwired: 11 in]
      n206 = call "BRig_dataExp_T_Reward_max_L.vi"() -> ("output_T_Reward_max_L"=w237:i32)  [unwired: 11 in]
      n207 = call "BRig_dataExp_T_Reward_max_R.vi"() -> ("output_T_Reward_max_R"=w236:i32)  [unwired: 11 in]
      n208 = call "BRig_dataExp_T_Reward_step_L.vi"() -> ("output_T_Reward_step_L"=w235:i32)  [unwired: 11 in]
      n209 = call "BRig_dataExp_T_Reward_step_R.vi"() -> ("output_T_Reward_step_R"=w234:i32)  [unwired: 11 in]
      n210 = call "BRig_dataExp_T_RewardPost.vi"() -> ("output_T_RewardPost"=w233:i32)  [unwired: 11 in]
      n211 = call "BRig_dataExp_T_Wrong.vi"() -> ("output_T_Wrong"=w232:i32)  [unwired: 11 in]
      n212 = call "BRig_dataExp_T_Timeout.vi"() -> ("output_T_Timeout"=w231:i32)  [unwired: 11 in]
      n213 = Index Array(array=w177, index #1=w251, index #2=w250, index #3=w249, index #4=w248, index #5=w247, index #6=w246, index #7=w245, index #8=w244, index #9=w243, index #10=w242, index #11=w241, index #12=w240, index #13=w239, index #14=w238, index #15=w237, index #16=w236, index #17=w235, index #18=w234, index #19=w233, index #20=w232, index #21=w231) -> (element #1=w230:u16, element #2=w229:u16, element #3=w228:u16, element #4=w227:u16, element #5=w226:u16, element #6=w225:u16, element #7=w224:u16, element #8=w223:u16, element #9=w222:u16, element #10=w221:u16, element #11=w220:u16, element #12=w219:u16, element #13=w218:u16, element #14=w217:u16, element #15=w216:u16, element #16=w215:u16, element #17=w214:u16, element #18=w213:u16, element #19=w212:u16, element #20=w211:u16, element #21=w210:u16)
      n214 = local write "T_ENL_min"(w230) -> ()
      n215 = local write "T_ENL_max"(w229) -> ()
      n216 = local write "T_ENL_step"(w228) -> ()
      n217 = local write "T_ENLPenalty"(w227) -> ()
      n218 = local write "T_Cue_Audio_min"(w226) -> ()
      n219 = local write "T_Cue_Audio_max"(w225) -> ()
      n220 = local write "T_Cue_Audio_step"(w224) -> ()
      n221 = local write "T_Cue_LED_min"(w223) -> ()
      n222 = local write "T_Cue_LED_max"(w222) -> ()
      n223 = local write "T_Cue_LED_step"(w221) -> ()
      n224 = local write "T_CuePenalty"(w220) -> ()
      n225 = local write "Tcycle_Selection"(w219) -> ()
      n226 = local write "Tcycle_Reward_min_L"(w218) -> ()
      n227 = local write "Tcycle_Reward_min_R"(w217) -> ()
      n228 = local write "Tcycle_Reward_max_L"(w216) -> ()
      n229 = local write "Tcycle_Reward_max_R"(w215) -> ()
      n230 = local write "Tcycle_Reward_step_L"(w214) -> ()
      n231 = local write "Tcycle_Reward_step_R"(w213) -> ()
      n232 = local write "Tcycle_RewardPost"(w212) -> ()
      n233 = local write "Tcycle_Wrong"(w211) -> ()
      n234 = local write "Tcycle_Timeout"(w210) -> ()
    }
  }
  "output_dataExp" <- w3
